vi "UpdateJSONFile.vi"(0 "Event":variant) -> ()   [LabVIEW 2018]
uses:
  <vilib>/LVH/i3 JSON/i3-json.lvlib
  Global Variables.vi
  <vilib>/LVH/i3 JSON/JSON Generation/Append to Array Files/Append to Array - Object.vi
  <vilib>/LVH/i3 JSON/JSON Parsing/Get Object Parameter Files/Get Object Parameter - Object.vi
  <vilib>/LVH/i3 JSON/JSON Parsing/Get Array Value at Index Files/Get Array Value at Index - Object.vi
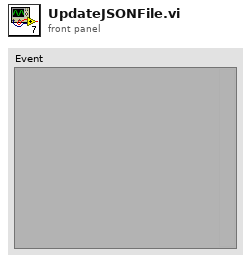
[diagram p1: front panel]
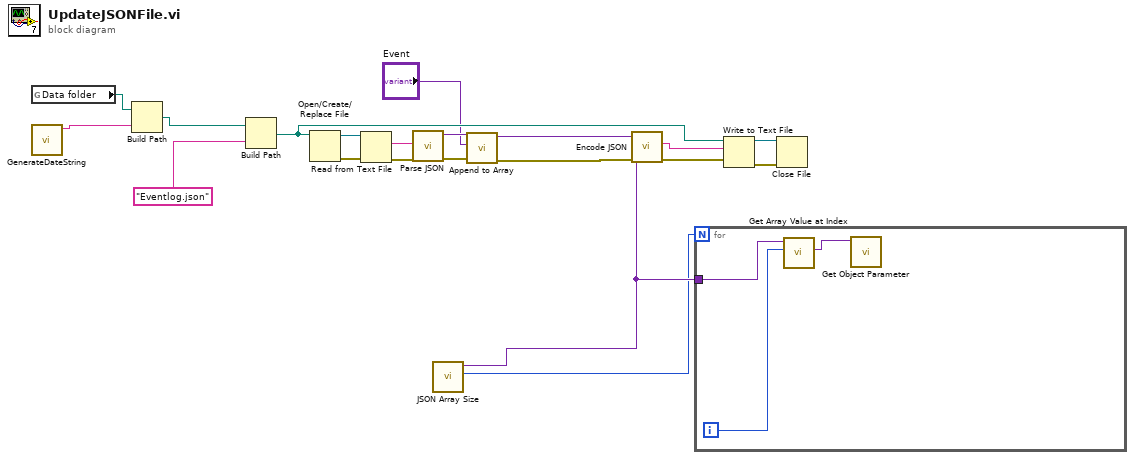
[diagram p0: block diagram]
diagram:
  n1 = global read "Global Variables.vi" "Data folder"() -> (w15:path)
  n2 = call "GenerateDateString.vi"() -> ("String"=w16:string)  [unwired: 11 in]
  n3 = Build Path(base path=w15, name or relative path=w16) -> (appended path=w14:path)
  n4 = Build Path(base path=w14, name or relative path="Eventlog.json" ("string")) -> (appended path=w12:path)
  n5 = Open/Create/Replace File(file path (use dialog)=w12) -> (refnum out=w11:refnum<file>, error out=w5:errorcluster)  [unwired: 5 in, 1 out]
  n6 = Read from Text File(file (use dialog)=w11, error in=w5) -> (text=w9:string, error out=w10:errorcluster)  [unwired: 2 in, 2 out]
  n7 = call <vilib>:"Parse JSON.vi"("error in (no error)"=w10, "JSON String"=w9) -> ("error out"=w8:errorcluster, "JSON Tree"=w7:variant)  [unwired: 6 in, 2 out]
  n8 = call-poly <vilib>:"Append to Array.vi"("error in (no error)"=w8, "JSON Object"="Event", "JSON Tree in (JSON Array)"=w7) -> ("error out"=w4:errorcluster, "JSON Tree out (JSON Array)"=w2:variant)  [unwired: 7 in]
  n9 = call <vilib>:"JSON Array Size.vi"("JSON Tree In (JSON Array)"=w2) -> ("Array Size"=w1:i32)  [unwired: 8 in, 2 out]
  n10 = call <vilib>:"Encode JSON.vi"("error in (no error)"=w4, "JSON Tree"=w2) -> ("error out"=w19:errorcluster, "String"=w3:string)  [unwired: 4 in]
  n11 = for {
    N: w1 -> [_]
    tunnel: w2 -> [w22]
    i -> [w21]
    n12 = call-poly <vilib>:"Get Array Value at Index.vi"("Index"=w21, "JSON Tree In (JSON Array)"=w22) -> ("JSON Object"=w20:variant)  [unwired: 6 in, 3 out]
    n13 = call-poly <vilib>:"Get Object Parameter.vi"("JSON Tree In (JSON Object)"=w20) -> ()  [unwired: 7 in, 4 out]
  }
  n14 = Write to Text File(file (use dialog)=w12, text=w3, error in=w19) -> (refnum out=w17:refnum<file>, error out=w18:errorcluster)  [unwired: 1 in, 1 out]
  n15 = Close File(refnum=w17, error in=w18) -> ()  [unwired: 2 out]
